vi "torque -- read field sweep file V1.vi"(0 "folder path":path=path "C:/Users/224586/Downloads/arkady/Torque-Jun2013/rotationset5/30K", 1 "filename":string="30K_0D_011_061413.dat") -> (16 "torque -- hash value":T1={"time (sec) array"=[], "temperature (K) array"=[], "SRS Vx (V) array"=[], "field (T) array"=[], "filename"="30K_0D_011_061413.dat", "time OK?"=FALSE, "temperature OK?"=FALSE, "SRS OK?"=FALSE, "FIELD OK?"=FALSE}, 17 "OK?":bool=TRUE)   [LabVIEW 2015]
uses:
  torque -- hash value.ctl
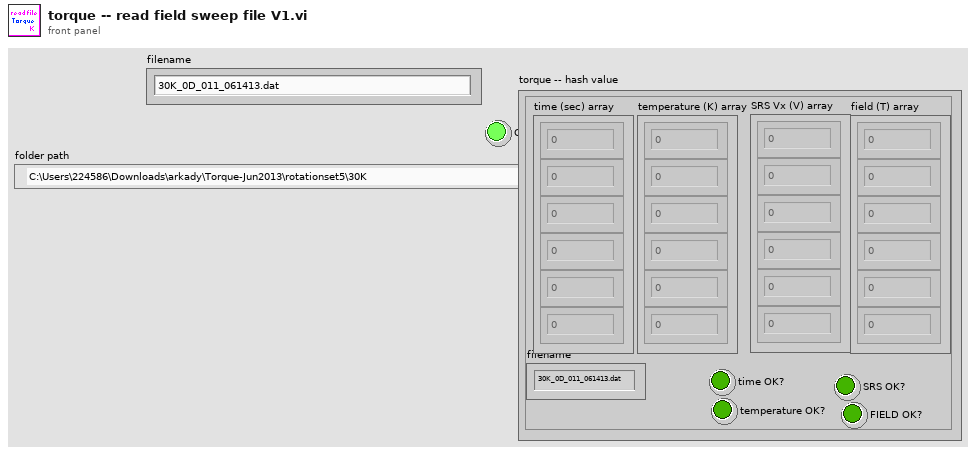
[diagram p1: front panel]
types:
  T1 = typedef "torque -- hash value.ctl" = cluster{"time (sec) array":dbl[], "temperature (K) array":dbl[], "SRS Vx (V) array":dbl[], "field (T) array":dbl[], "filename":string, "time OK?":bool, "temperature OK?":bool, "SRS OK?":bool, "FIELD OK?":bool}
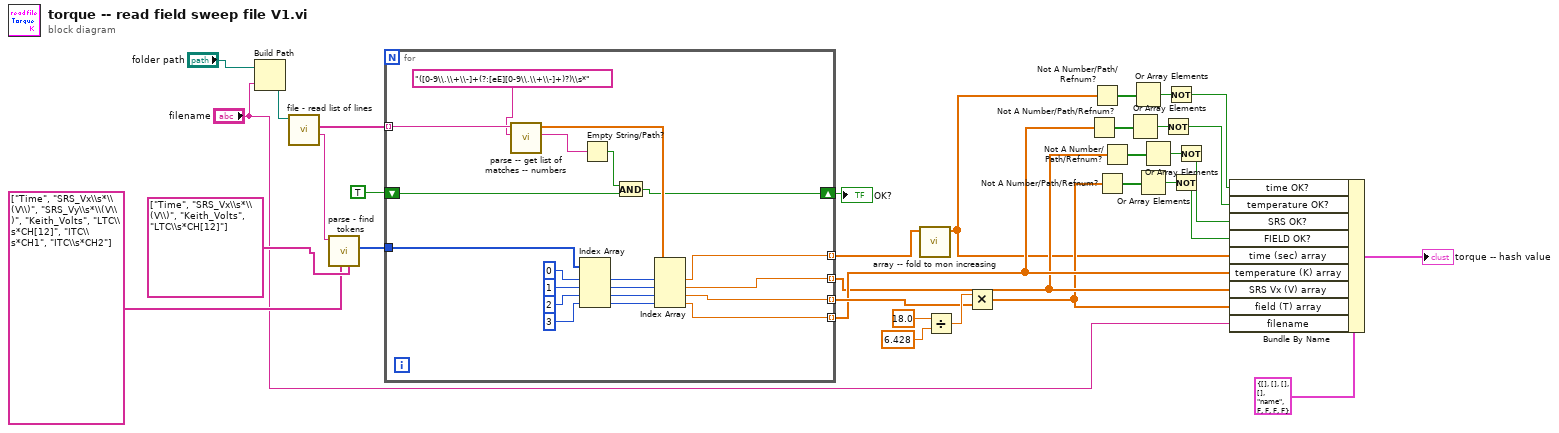
[diagram p0: block diagram]
diagram:
  n1 = Build Path(base path="folder path", name or relative path="filename") -> (appended path=w19:path)
  n2 = call "file - read list of lines.vi"("file path"=w19) -> ("first line"=w27:string, "list of lines"=w28:string[])  [unwired: 9 in]
  n3 = call "parse - find tokens.vi"("tokens wanted"=string[] ["Time", "SRS_Vx\\s*\\(V\\)", "Keith_Volts", "LTC\\s*CH[12]"], "all tokens"=string[] ["Time", "SRS_Vx\\s*\\(V\\)", "SRS_Vy\\s*\\(V\\)", "Keith_Volts", "LTC\\s*CH[12]", "ITC\\s*CH1", "ITC\\s*CH2"], "line"=w27) -> ("token indices"=w29:i32[])  [unwired: 8 in]
  n4 = for {
    tunnel: w28 -> [w53] mode=indexing
    shift-right: [w43] -> w32
    shift-left: TRUE -> [w44]
    tunnel: [w42] -> w2 mode=indexing
    tunnel: [w41] -> w6 mode=indexing
    tunnel: [w40] -> w23 mode=indexing
    tunnel: [w39] -> w9 mode=indexing
    tunnel: w29 -> [w37]
    n5 = call "parse -- get list of matches -- numbers.vi"("regexp"="([0-9\\.\\+\\-]+(?:[eE][0-9\\.\\+\\-]+)?)\\s*", "string"=w53) -> ("after match"=w46:string, "Array of numbers"=w51:dbl[])  [unwired: 6 in, 2 out]
    n6 = Index Array(array=w37, index #1=0 ("index"), index #2=1 ("index"), index #3=2 ("index"), index #4=3 ("index")) -> (element #1=w38:i32, element #2=w36:i32, element #3=w35:i32, element #4=w34:i32)
    n7 = Empty String/Path?(string/path=w46) -> (empty?=w45:bool)
    n8 = And(x=w45, y=w44) -> (x .and. y?=w43:bool)
    n9 = Index Array(array=w51, index #1=w38, index #2=w36, index #3=w35, index #4=w34) -> (element #1=w42:dbl, element #2=w41:dbl, element #3=w40:dbl, element #4=w39:dbl)
  }
  "OK?" <- w32
  n10 = call "array -- fold to mon increasing.vi"("Array"=w2) -> ("Array out"=w1:dbl[])  [unwired: 10 in]
  n11 = Divide(x=18.0, y=6.428 ("x")) -> (x/y=w24:dbl)
  n12 = Multiply(x=w24, y=w23) -> (x*y=w4:dbl[])
  n13 = Not A Number/Path/Refnum?(number/path/refnum=w9) -> (NaN/Path/Refnum?=w13:bool[])
  n14 = Not A Number/Path/Refnum?(number/path/refnum=w1) -> (NaN/Path/Refnum?=w17:bool[])
  n15 = Not A Number/Path/Refnum?(number/path/refnum=w4) -> (NaN/Path/Refnum?=w11:bool[])
  n16 = Not A Number/Path/Refnum?(number/path/refnum=w6) -> (NaN/Path/Refnum?=w15:bool[])
  n17 = Or Array Elements(Boolean array=w13) -> (logical OR=w12:bool)
  n18 = Or Array Elements(Boolean array=w17) -> (logical OR=w16:bool)
  n19 = Or Array Elements(Boolean array=w11) -> (logical OR=w10:bool)
  n20 = Or Array Elements(Boolean array=w15) -> (logical OR=w14:bool)
  n21 = Not(x=w12) -> (.not. x?=w7:bool)
  n22 = Not(x=w16) -> (.not. x?=w8:bool)
  n23 = Not(x=w10) -> (.not. x?=w3:bool)
  n24 = Not(x=w14) -> (.not. x?=w5:bool)
  n25 = Bundle By Name(cluster=T1 {"time (sec) array"=[], "temperature (K) array"=[], "SRS Vx (V) array"=[], "field (T) array"=[], "filename"="name", "time OK?"=FALSE, "temperature OK?"=FALSE, "SRS OK?"=FALSE, "FIELD OK?"=FALSE} ("torque -- hash value"), "time OK?"=w8, "temperature OK?"=w7, "SRS OK?"=w5, "FIELD OK?"=w3, "time (sec) array"=w1, "temperature (K) array"=w9, "SRS Vx (V) array"=w6, "field (T) array"=w4, "filename"="filename") -> (→"torque -- hash value":T1)
